vi "Write File Transfer Behavior.lvclass.vi"(8 "error in (no error)":errorcluster, 10 "RT Management.lvlib:File Transfer Behavior.lvclass":refnum<class "File Transfer Behavior.lvclass">, 11 "[Test Case] File or directory exists in":refnum<class "[Test Case] File or directory exists.lvclass">) -> (0 "error out":errorcluster, 3 "[Test Case] File or directory exists out":refnum<class "[Test Case] File or directory exists.lvclass">)   [LabVIEW 2015, in "Tests.lvlib" / "[Test Case] File or directory exists.lvclass"]
uses:
  [Test Case] File or directory exists.lvclass
  classes/File Transfer Behavior/File Transfer Behavior.lvclass
  [Test Case] File or directory exists.lvclass/[Test Case] File or directory exists.ctl
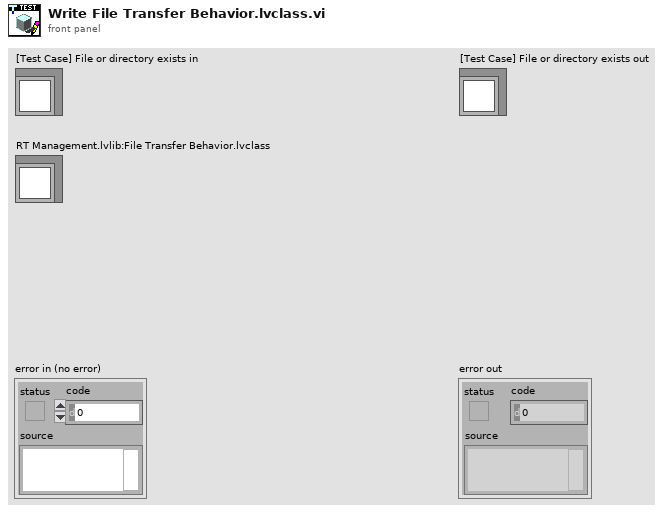
[diagram p1: front panel]
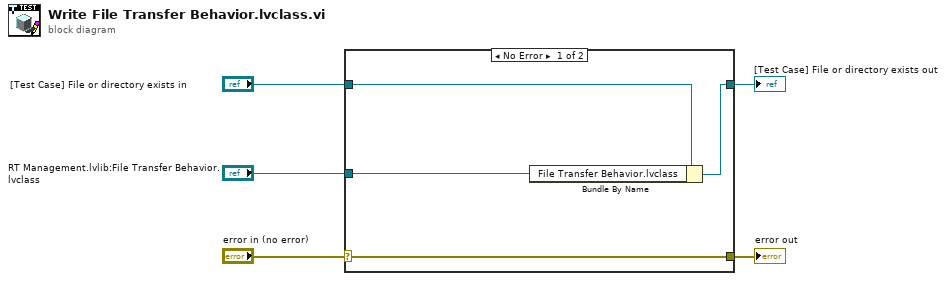
[diagram p0: block diagram]
diagram:
  n1 = case shown="No Error" "error in (no error)" {
    selector: "error in (no error)" -> [w9 w10]
    tunnel: [w9 w10] -> w4
    tunnel: [w7 w11] -> w2
    tunnel: "[Test Case] File or directory exists in" -> [w8 w11]
    tunnel: "RT Management.lvlib:File Transfer Behavior.lvclass" -> [w6 _]
    frame No Error {
      n2 = Bundle By Name(cluster=w8, "File Transfer Behavior.lvclass"=w6) -> (w7:refnum<class "[Test Case] File or directory exists.lvclass">)
    }
    frame Error {
    }
  }
  "error out" <- w4
  "[Test Case] File or directory exists out" <- w2
